vi "Set Waveform Streams for Data Event.vi"   [LabVIEW 2020, in "NI_VS Waveform Streaming Interface.lvlib"]
doc: "Updates the event registration to apply to the waveform stream specifications you specify. This VI is useful for changing the waveforms for which you want to receive data events without stopping the current event-handling routine and re-registering for waveform-data events."
uses:
  <vilib>/NI VeriStand/Execution/WaveformStreaming/NI_VS Waveform Streaming Interface.lvlib
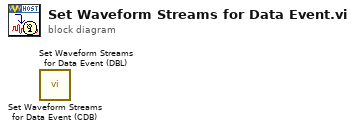
[diagram p0: block diagram]
diagram:
  n1 = call <vilib>:"Set Waveform Streams for Data Event (CDB).vi"() -> ()  [unwired: 10 in, 2 out]
  n2 = call <vilib>:"Set Waveform Streams for Data Event (DBL).vi"() -> ()  [unwired: 10 in, 2 out]
